vi "Stop RPC Engine Loops.vi"(8 "error in (no error)":errorcluster) -> (0 "error out":errorcluster)   [LabVIEW 2016, in "JSONRPC Server.lvclass"]
uses:
  JSONRPC Server.lvclass
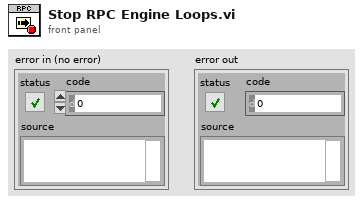
[diagram p1: front panel]
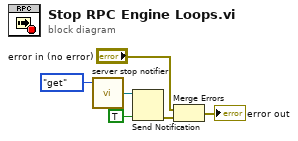
[diagram p0: block diagram]
diagram:
  n1 = call "server stop notifier.vi"("action"=enum16{"get", "set"}."get") -> ("notifier out"=w5:refnum<notifier>)  [unwired: 2 in]
  n2 = Send Notification(notification=TRUE, notifier=w5) -> (error out=w3:errorcluster)  [unwired: 1 in, 1 out]
  n3 = Merge Errors("error in (no error)", w3) -> (→"error out":errorcluster)
